vi "Do.vi"(8 "error in (no error)":errorcluster, 10 "Actor in":refnum<class "Actor.lvclass">, 11 "Set f0 MSG":refnum<class "Set f0 MSG.lvclass">) -> (0 "error out":errorcluster, 2 "Actor out":refnum<class "Actor.lvclass">)   [LabVIEW 2014, in "ePAS Library.lvlib" / "Set f0 MSG.lvclass"]
doc: "(<B>Filename</B>: Actor Framework.lvlib:Message.lvclass:Do.vi)\n\nDefines what a message does when it is received by an actor. Generally, a message instructs an actor to invoke one of its methods. By default, this method does nothing. A child class must override it to define behavior. Create a child class by using the Actor Framework Message Maker dialog box."
uses:
  Set f0 MSG.lvclass
  <vilib>/ActorFramework/Actor/Actor.lvclass
  Set f0 MSG.lvclass/Set f0 MSG.ctl
  Instr Actor.lvclass
  PAS/Commands/Change PAS Laser Frequency/Change Laser Frequency.lvclass
  PAS/Commands/Change PAS Laser Frequency/Change Laser Frequency.lvclass/Change Laser Frequency.ctl
  Controller/Messages/Update CVT/Update CVT Data.lvclass
  Controller/Messages/Update CVT/Update CVT Data.lvclass/Update CVT Data.ctl
  Controller/Messages/Update CVT/Write tag.vi
  Controller/Messages/Update CVT/Write Data.vi
  Controller/Messages/Update CVT/Write Group.vi
  reusable/Command/Command.lvclass
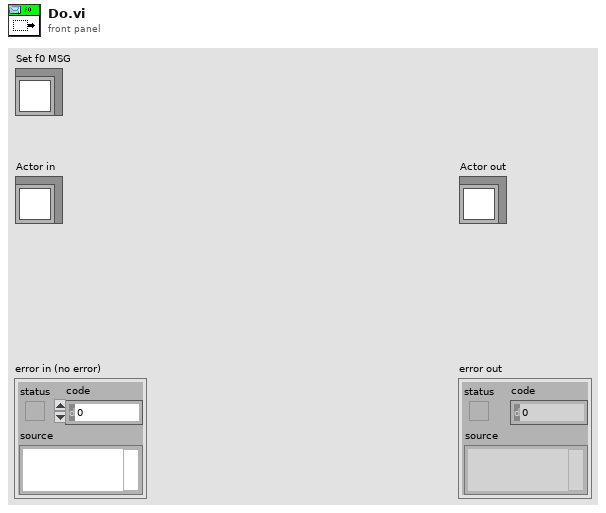
[diagram p1: front panel]
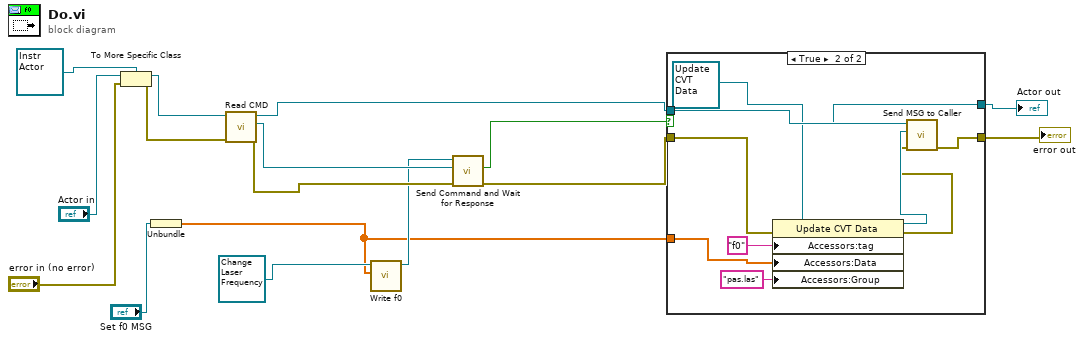
[diagram p0: block diagram]
diagram:
  n1 = To More Specific Class(target class=refnum<class "Instr Actor.lvclass"> refnum ("Instrument Lib:Instr"), reference="Actor in", error in="error in (no error)") -> (specific class reference=w14:refnum<class "Instr Actor.lvclass">, error out=w13:errorcluster)
  n2 = Unbundle("Set f0 MSG") -> (w6:sgl[])
  n3 = call "Read CMD.vi"("error in (no error)"=w13, "Instr Actor in"=w14) -> ("error out"=w8:errorcluster, "CMD"=w9:refnum<queue>, "Instr Actor out"=w5:refnum<class "Instr Actor.lvclass">)  [unwired: 7 in]
  n4 = call "Write f0.vi"("f0"=w6, "Change Laser Frequency in"=refnum<class "Change Laser Frequency.lvclass"> refnum ("Change Laser Frequency.lvclass")) -> ("Change Laser Frequency out"=w7:refnum<class "Change Laser Frequency.lvclass">)  [unwired: 8 in, 1 out]
  n5 = call "Send Command and Wait for Response.vi"("error in"=w8, "cmd queue"=w9, "CMD in"=w7) -> ("error out"=w3:errorcluster, "cmd good?"=w4:bool)  [unwired: 6 in, 1 out]
  n6 = case shown="True" w4 {
    tunnel: w5 -> [w18 w28]
    tunnel: [w18 w27] -> w1
    tunnel: w3 -> [w17 w23]
    tunnel: [w17 w26] -> w2
    tunnel: w6 -> [_ w21]
    frame False {
    }
    frame True {
      n7 = property class="Update CVT Data"(reference=refnum<class "Update CVT Data.lvclass"> refnum ("Controller.lvlib:Update CVT Data"), error in=w23, "Accessors:tag"="f0" ("Key"), "Accessors:Data"=w21, "Accessors:Group"="pas.las" ("Group")) -> (reference out=w24:refnum<class "Update CVT Data.lvclass">, error out=w22:errorcluster)
      n8 = call "Send MSG to Caller.vi"("error in"=w22, "Message"=w24, "Instr in"=w28) -> ("error out"=w26:errorcluster, "Instr out"=w27:refnum<class "Instr Actor.lvclass">)  [unwired: 7 in]
    }
  }
  "error out" <- w2
  "Actor out" <- w1
